vi "tab control refresh.vi"(4 "name string":string, 6 "C header file directory":path, 8 "error in":errorcluster, 9 "output file string":string, 10 "input file string":string, 11 "VI reference":refnum<vi>) -> (0 "error out":errorcluster)   [LabVIEW 2013, in "Shared Memory editor node.lvclass"]
doc: "***TODO***\n\n<B>Input Parameters</B>\n\n<B>error in</B> describes error conditions that occur before this node runs. This input provides standard error in functionality.\n\n<B>write directory</B> ***TODO***write directory\n\n<B>read directory</B> ***TODO***read directory\n\n<B>VI reference</B> ***TODO***VI reference\n\n<B>Output Parameters</B>\n\n<B>error out</B> contains error information. This output provides standard error out functionality."
uses:
  Shared Memory editor node.lvclass
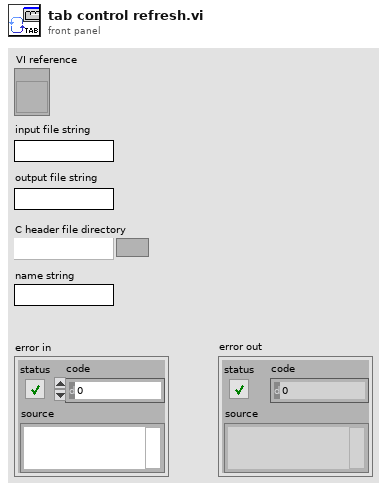
[diagram p1: front panel]
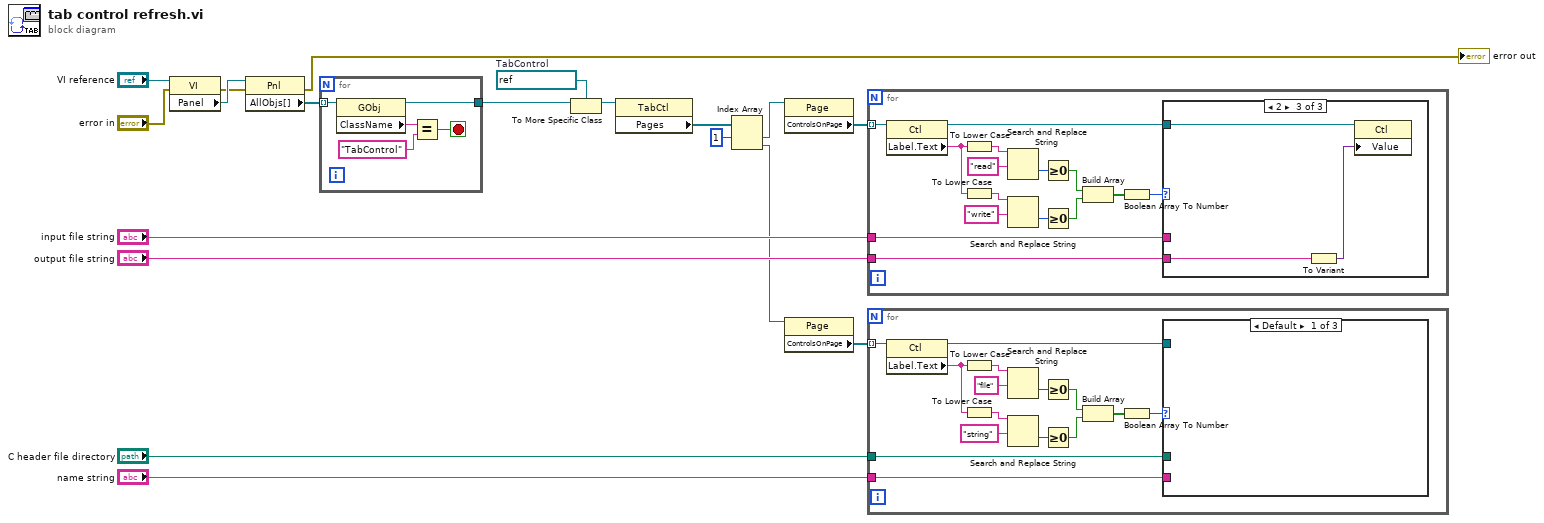
[diagram p0: block diagram]
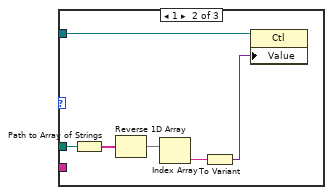
[diagram p2: hidden frame]
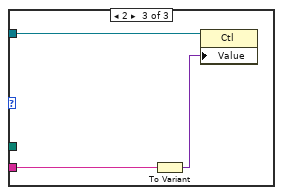
[diagram p3: hidden frame]
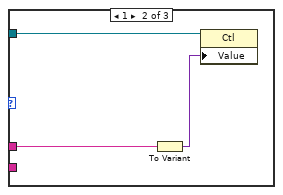
[diagram p5: hidden frame]
diagram:
  w14 = refnum<vi> refnum  # TabControl
  n1 = property class="VI"(reference="VI reference", error in="error in") -> (error out=w10:errorcluster, "Panel"=w12:refnum<vi>)  [unwired: 1 out]
  n2 = property class="Pnl"(reference=w12, error in=w10) -> (error out=→"error out":errorcluster, "AllObjs[]"=w11:refnum<vi>[])  [unwired: 1 out]
  n3 = for {
    tunnel: w11 -> [w24] mode=indexing
    tunnel: [w23] -> w13
    stop <- w20 stop-if-true
    n4 = property class="GObj"(reference=w24) -> (reference out=w23:refnum<vi>, "ClassName"=w21:string)  [unwired: 1 in, 1 out]
    n5 = Equal?(x=w21, y="TabControl") -> (x = y?=w20:bool)
  }
  n6 = To More Specific Class(target class=w14, reference=w13) -> (specific class reference=w15:refnum<vi>)  [unwired: 1 in, 1 out]
  n7 = property class="TabCtl"(reference=w15) -> ("Pages"=w16:refnum<vi>[])  [unwired: 1 in, 2 out]
  n8 = Index Array(array=w16, index #1=1 ("index")) -> (element #1=w18:refnum<vi>, element #2=w1:refnum<vi>)  [unwired: 1 in]
  n9 = property class="Page"(reference=w18) -> ("ControlsOnPage"=w19:refnum<vi>[])  [unwired: 1 in, 2 out]
  n10 = property class="Page"(reference=w1) -> ("ControlsOnPage"=w4:refnum<vi>[])  [unwired: 1 in, 2 out]
  n11 = for {
    tunnel: w19 -> [w39] mode=indexing
    tunnel: "input file string" -> [w26]
    tunnel: "output file string" -> [w25]
    n12 = property class="Ctl"(reference=w39) -> (reference out=w38:refnum<vi>, "Label.Text"=w33:string)  [unwired: 1 in, 1 out]
    n13 = To Lower Case(string=w33) -> (all lower case string=w37:string)
    n14 = To Lower Case(string=w33) -> (all lower case string=w34:string)
    n15 = Search and Replace String(input string=w37, search string="read") -> (offset past replacement=w32:i32)  [unwired: 6 in, 3 out]
    n16 = Search and Replace String(input string=w34, search string="write") -> (offset past replacement=w31:i32)  [unwired: 6 in, 3 out]
    n17 = Greater Or Equal To 0?(x=w32) -> (x >= 0?=w30:bool)
    n18 = Greater Or Equal To 0?(x=w31) -> (x >= 0?=w29:bool)
    n19 = Build Array(w30, w29) -> (w28:bool[])
    n20 = Boolean Array To Number(Boolean array=w28) -> (number=w27:u32)
    n21 = case shown="2" w27 {
      tunnel: w38 -> [_ w42 w45]
      tunnel: w26 -> [_ w40 _]
      tunnel: w25 -> [_ _ w43]
      frame Default {
      }
      frame 1 {
        n22 = To Variant(anything=w40) -> (Variant=w41:variant)
        n23 = property class="Ctl"(reference=w42, "Value"=w41) -> ()  [unwired: 1 in, 2 out]
      }
      frame 2 {
        n24 = To Variant(anything=w43) -> (Variant=w44:variant)
        n25 = property class="Ctl"(reference=w45, "Value"=w44) -> ()  [unwired: 1 in, 2 out]
      }
    }
  }
  n26 = for {
    tunnel: w4 -> [w60] mode=indexing
    tunnel: "C header file directory" -> [w47]
    tunnel: "name string" -> [w46]
    n27 = property class="Ctl"(reference=w60) -> (reference out=w59:refnum<vi>, "Label.Text"=w54:string)  [unwired: 1 in, 1 out]
    n28 = To Lower Case(string=w54) -> (all lower case string=w58:string)
    n29 = To Lower Case(string=w54) -> (all lower case string=w55:string)
    n30 = Search and Replace String(input string=w58, search string="file") -> (offset past replacement=w53:i32)  [unwired: 6 in, 3 out]
    n31 = Search and Replace String(input string=w55, search string="string") -> (offset past replacement=w52:i32)  [unwired: 6 in, 3 out]
    n32 = Greater Or Equal To 0?(x=w53) -> (x >= 0?=w51:bool)
    n33 = Greater Or Equal To 0?(x=w52) -> (x >= 0?=w50:bool)
    n34 = Build Array(w51, w50) -> (w49:bool[])
    n35 = Boolean Array To Number(Boolean array=w49) -> (number=w48:u32)
    n36 = case shown="Default" w48 {
      tunnel: w59 -> [_ w66 w69]
      tunnel: w47 -> [_ w64 _]
      tunnel: w46 -> [_ _ w67]
      frame Default {
      }
      frame 1 {
        n37 = Path to Array of Strings(0:w64) -> (2:w63:string[])  [unwired: 1 out]
        n38 = Reverse 1D Array(array=w63) -> (reversed array=w62:string[])
        n39 = Index Array(array=w62) -> (element=w61:string)  [unwired: 1 in]
        n40 = To Variant(anything=w61) -> (Variant=w65:variant)
        n41 = property class="Ctl"(reference=w66, "Value"=w65) -> ()  [unwired: 1 in, 2 out]
      }
      frame 2 {
        n42 = To Variant(anything=w67) -> (Variant=w68:variant)
        n43 = property class="Ctl"(reference=w69, "Value"=w68) -> ()  [unwired: 1 in, 2 out]
      }
    }
  }
